vi "Model - Get Stop.vi"(8 "error in (no error)":errorcluster, 11 "View Model":T1) -> (0 "error out":errorcluster, 2 "Stop":bool, 3 "View Model":T1)   [LabVIEW 2017]
doc: "Get actual Stop Value from DVR"
uses:
  Controls/View Model.ctl
  Controls/Shared Model.ctl
  Error Handler/Controls/Error Model.ctl
  Error Handler/Controls/Error Message.ctl
  Error Handler/Controls/Error Level.ctl
  Configuration/Controls/Database Model.ctl
  Configuration/Controls/Database Message.ctl
  Configuration/Controls/Database Command.ctl
  Configuration/Controls/Database Overhead.ctl
  Configuration/Controls/Database Status.ctl
  Configuration/Controls/Database Record.ctl
  Configuration/Controls/Database - Rule Record.ctl
  Controller/Controls/CNTRLR - Wash Step.ctl
  Controller/Controls/CNTRLR - Position.ctl
  Controller/Controls/CNTRLR - Model.ctl
  Controller/Controls/CNTRLR - Message.ctl
  Controller/Controls/CNTRLR - Command.ctl
  Controller/Controls/CNTRLR - Overhead.ctl
  Controller/Controls/CNTRLR - State.ctl
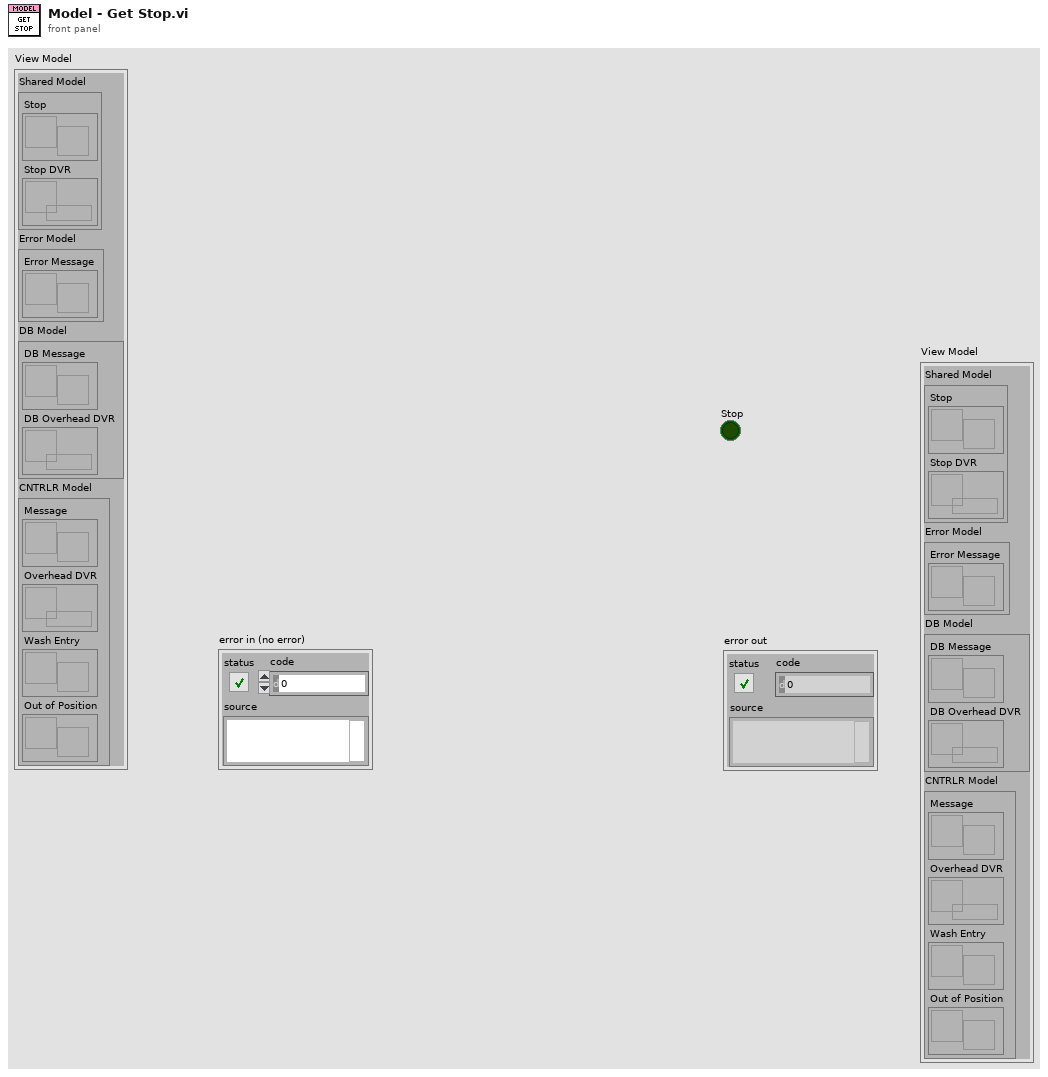
[diagram p1: front panel]
types:
  T1 = typedef "View Model.ctl" = cluster{"Shared Model":T2, "Error Model":T3, "DB Model":T4, "CNTRLR Model":T5}
  T2 = typedef "Shared Model.ctl" = cluster{"Stop":refnum<user-event>, "Stop DVR":refnum<data-value>}
  T3 = typedef "Error Model.ctl" = cluster{"Error Message":refnum<user-event>}
  T4 = typedef "Database Model.ctl" = cluster{"DB Message":refnum<user-event>, "DB Overhead DVR":refnum<data-value>}
  T5 = typedef "CNTRLR - Model.ctl" = cluster{"Message":refnum<user-event>, "Overhead DVR":refnum<data-value>, "Wash Entry":refnum<user-event>, "Out of Position":refnum<user-event>}
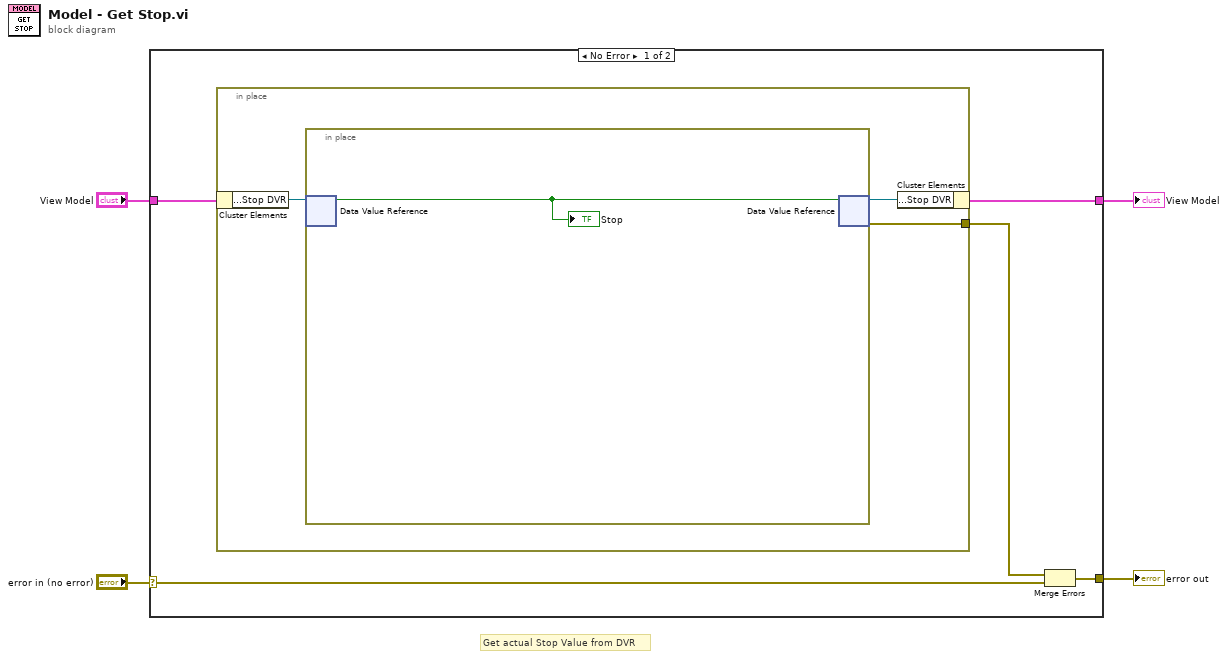
[diagram p0: block diagram]
diagram:
  # "Get actual Stop Value from DVR"
  n1 = case shown="No Error" "error in (no error)" {
    selector: "error in (no error)" -> [w7 w15]
    tunnel: [w5 w15] -> w3
    tunnel: "View Model" -> [w9 w14]
    tunnel: [w8 w14] -> w1
    frame No Error {
      n2 = in-place {
        in-place-border: [w10] -> w6
        n3 = in-place-cluster #1(w9) -> ("Shared Model.Stop DVR"=w12:refnum<data-value>)
        n4 = in-place {
          n5 = in-place-dvr #2(w12) -> (w13:bool)  [unwired: 1 out]
          "Stop" <- w13
          n6 = in-place-dvr #2(w13) -> (w11:refnum<data-value>, w10:errorcluster)
        }
        n7 = in-place-cluster #1("Shared Model.Stop DVR"=w11) -> (w8:T1)
      }
      n8 = Merge Errors(w6, w7) -> (w5:errorcluster)
    }
    frame Error {
      # "If any Error occurred do nothing"
    }
  }
  "error out" <- w3
  "View Model" <- w1
